vi "API - Delete Conflicting Mappings.vi"(8 "error in (no error)":errorcluster, 10 "Channels":T1[](array[typedef]) {"Destination Ref" format="%.0x"}, 11 "Rx Section Ref In":T2 format="%.0x") -> (0 "error out":errorcluster, 3 "Rx Section Ref Out":T2 format="%.0x")   [LabVIEW 2016, in "UDP-Custom-Device System Explorer.lvlib"]
uses:
  UDP-Custom-Device System Explorer.lvlib
  <vilib>/NI Veristand/Custom Device API/Custom Device Item Ref.ctl
  TypeDef - Channel Data.ctl
  Shared/DataTypes.ctl
  NationalInstruments.VeriStand.SystemDefinitionAPI
  <vilib>/NI VeriStand/Custom Device API/Custom Device API.lvlib
  Shared/UDP-Custom-Device Shared.lvlib
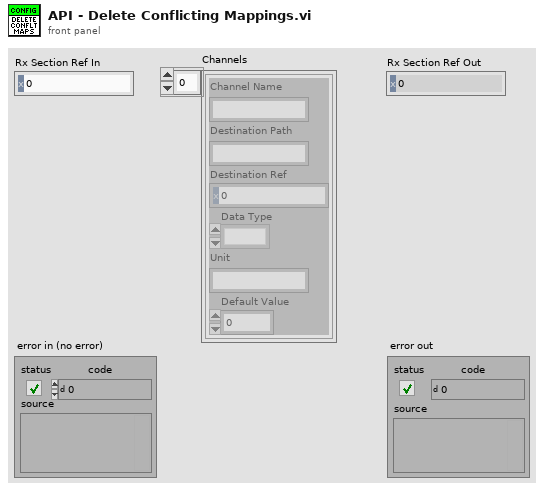
[diagram p1: front panel]
types:
  T1 = typedef "UDP-Custom-Device System Explorer.lvlib/TypeDef - Channel Data.ctl" = cluster{"Channel Name":string, "Destination Path":string, "Destination Ref":T2, "Data Type":T3, "Unit":string, "Default Value":dbl}
  T2 = typedef "Custom Device API.lvlib/Custom Device Item Ref.ctl" = u64
  T3 = typedef "UDP-Custom-Device Shared.lvlib/DataTypes.ctl" = enum16{""}
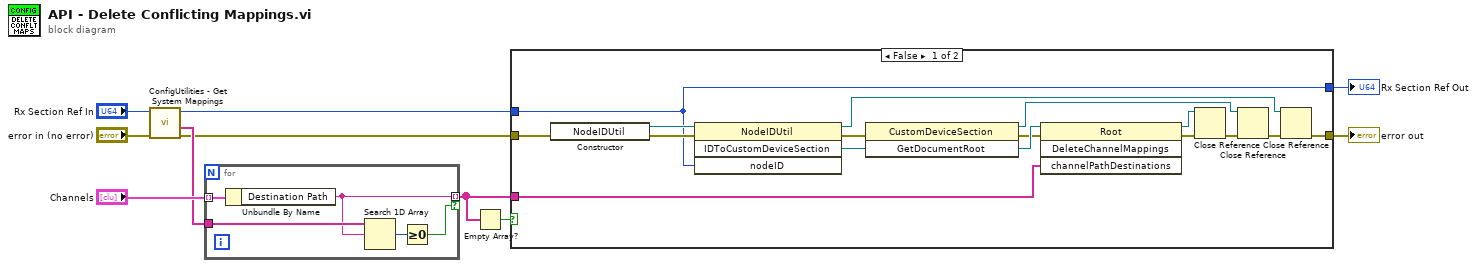
[diagram p0: block diagram]
diagram:
  n1 = call "ConfigUtilities - Get System Mappings.vi"("error in (no error)"="error in (no error)", "Item Ref in"="Rx Section Ref In") -> ("error out"=w3:errorcluster, "Channel Path Destinations"=w7:string[], "Item Ref out"=w4:T2)  [unwired: 6 in, 1 out]
  n2 = for {
    tunnel: "Channels" -> [w15] mode=indexing
    tunnel: w7 -> [w14]
    tunnel: [w12] -> w5 mode=indexing if=w11
    n3 = Unbundle By Name(w15) -> ("Destination Path"=w12:string)
    n4 = Search 1D Array(1D array=w14, element=w12) -> (index of element=w13:i32)  [unwired: 1 in]
    n5 = Greater Or Equal To 0?(x=w13) -> (x >= 0?=w11:bool)
  }
  n6 = Empty Array?(array=w5) -> (empty?=w6:bool)
  n7 = case shown="False" w6 {
    tunnel: w5 -> [w21 _]
    tunnel: w4 -> [w16 w33]
    tunnel: w3 -> [w22 w32]
    tunnel: [w16 w33] -> w1
    tunnel: [w23 w32] -> w2
    frame False {
      n8 = constructor class="NodeIDUtil"(error in=w22) -> (reference out=w27:refnum<k24>, error out=w26:errorcluster)  [unwired: 2 in, 1 out]
      n9 = invoke class="NodeIDUtil" method="IDToCustomDeviceSection"(reference=w27, error in=w26, "nodeID"=w16) -> (reference out=w17:refnum<k24>, error out=w25:errorcluster, "IDToCustomDeviceSection"=w28:refnum<k24>)  [unwired: 1 in, 1 out]
      n10 = invoke class="CustomDeviceSection" method="GetDocumentRoot"(reference=w28, error in=w25) -> (reference out=w18:refnum<k24>, error out=w20:errorcluster, "GetDocumentRoot"=w29:refnum<k24>)  [unwired: 1 in]
      n11 = invoke class="Root" method="DeleteChannelMappings"(reference=w29, error in=w20, "channelPathDestinations"=w21) -> (reference out=w19:refnum<k24>, error out=w24:errorcluster)  [unwired: 1 in, 2 out]
      n12 = Close Reference(reference=w19, error in (no error)=w24) -> (error out=w30:errorcluster)
      n13 = Close Reference(reference=w18, error in (no error)=w30) -> (error out=w31:errorcluster)
      n14 = Close Reference(reference=w17, error in (no error)=w31) -> (error out=w23:errorcluster)
    }
    frame True {
      # "No channels will attempt to be mapped to a channel with\nan existing mapping"
    }
  }
  "Rx Section Ref Out" <- w1
  "error out" <- w2
